vi "Ex8.vi"() -> ()   [LabVIEW 2019]
panel:
  in  "stop":bool
  out "Graphe déroulant":cluster{dbl, dbl, dbl}(graph)
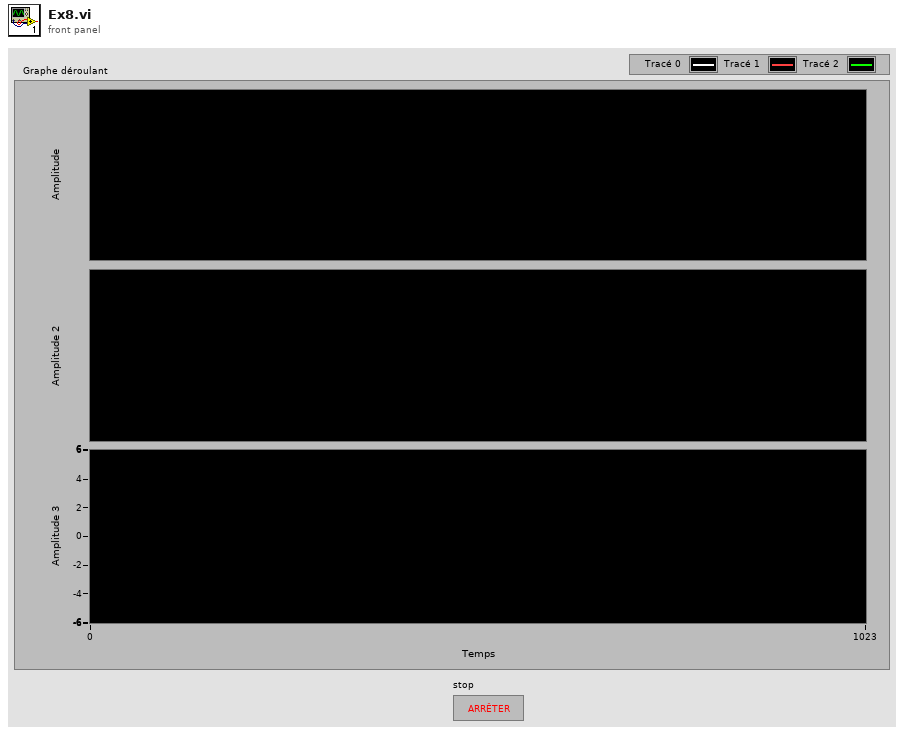
[diagram p1: front panel]
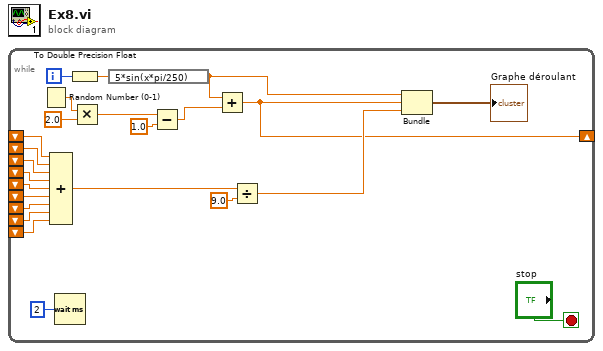
[diagram p0: block diagram]
diagram:
  n1 = while {
    shift-right: [w2] -> _
    shift-left: _ -> [w14]
    shift-left: _ -> [w13]
    shift-left: _ -> [w12]
    shift-left: _ -> [w11]
    shift-left: _ -> [w10]
    shift-left: _ -> [w9]
    shift-left: _ -> [w8]
    shift-left: _ -> [w7]
    shift-left: _ -> [w6]
    i -> [w21]
    stop <- "stop" stop-if-true
    n2 = Random Number (0-1)() -> (number: 0 to 1=w19:dbl)
    n3 = Compound Arithmetic op=ADD(w14, w13, w12, w11, w10, w9, w8, w7, w6) -> (w5:dbl)
    n4 = Wait (ms)(milliseconds to wait=u32 2 ("attente (ms)")) -> ()  [unwired: 1 out]
    n5 = To Double Precision Float(number=w21) -> (double precision float=w23:dbl)
    n6 = Multiply(x=w19, y=2.0) -> (x*y=w17:dbl)
    n7 = expression code="5*sin(x*pi/250)"(w23) -> (w15:dbl)
    n8 = Subtract(x=w17, y=1.0) -> (x-y=w1:dbl)
    n9 = Add(x=w15, y=w1) -> (x+y=w2:dbl)
    n10 = Divide(x=w5, y=9.0) -> (x/y=w3:dbl)
    n11 = Bundle(w15, w2, w3) -> (→"Graphe déroulant":cluster{dbl, dbl, dbl})  [unwired: 1 in]
  }
